vi "Trigger With SubVi.vi"() -> ()   [LabVIEW 2022 SP3]
uses:
  Keithley 24XX Sweep and Acquire Measurements Folder/Keithley 24XX.lvlib
  <instrlib>/Keithley 2182/Keithley 2182.lvlib
panel:
  in  "Enable Current Auto Range (T:Enable)":bool=TRUE
  in  "Current Manual Range (1.0)":dbl=1.0
  out "Measurements":dbl[](array[numeric])
  in  "Integration Rate (5)":dbl=5.0
  in  "Range Value (12)":dbl=12.0
  in  "Voltage Resolution (8)":i32=8
  in  "Measurement (0: Voltage Channel 1) 2":i32(ring) items=["Voltage Channel 1", "Voltage Channel 2", "Temperature Channel 1", "Temperature Channel 2"]
  in  "2182A":T1={"Baud Rate"=9600, "Parity"=0, "Data Bits"=8, "Stop Bits"=10, "Flow Control"=0, "VISA resource name"="SourceMeter2400"} {"Flow Control" items=["None", "XON/XOFF", "RTS/CTS", "XON/XOFF & RTS/CTS", "DTR/DSR", "XON/XOFF & DTR/DSR"]; "Stop Bits" items=["1.0"=10, "1.5"=15, "2.0"=20]; "Data Bits" items=["7"=7, "8"=8]; "Parity" items=["None", "Odd", "Even", "Mark", "Space"]; "Baud Rate" items=["300"=300, "600"=600, "1200"=1200, "2400"=2400, "4800"=4800, "9600"=9600, "19200"=19200]}
  in  "2400":T1={"Baud Rate"=9600, "Parity"=0, "Data Bits"=8, "Stop Bits"=10, "Flow Control"=0, "VISA resource name"="NanoVoltMeter2182"} {"Flow Control" items=["None", "XON/XOFF", "RTS/CTS", "XON/XOFF & RTS/CTS", "DTR/DSR", "XON/XOFF & DTR/DSR"]; "Stop Bits" items=["1.0"=10, "1.5"=15, "2.0"=20]; "Data Bits" items=["7"=7, "8"=8]; "Parity" items=["None", "Odd", "Even", "Mark", "Space"]; "Baud Rate" items=["300"=300, "600"=600, "1200"=1200, "2400"=2400, "4800"=4800, "9600"=9600, "19200"=19200]}
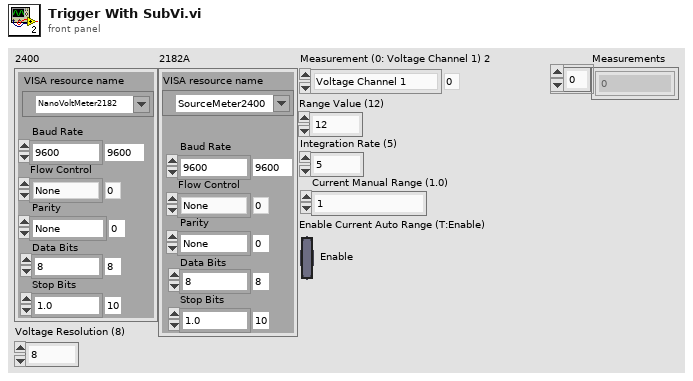
[diagram p1: front panel]
types:
  T1 = cluster{"Baud Rate":u32, "Parity":u16, "Data Bits":u16, "Stop Bits":u16, "Flow Control":u16, "VISA resource name":refnum<visa-resource-name>}
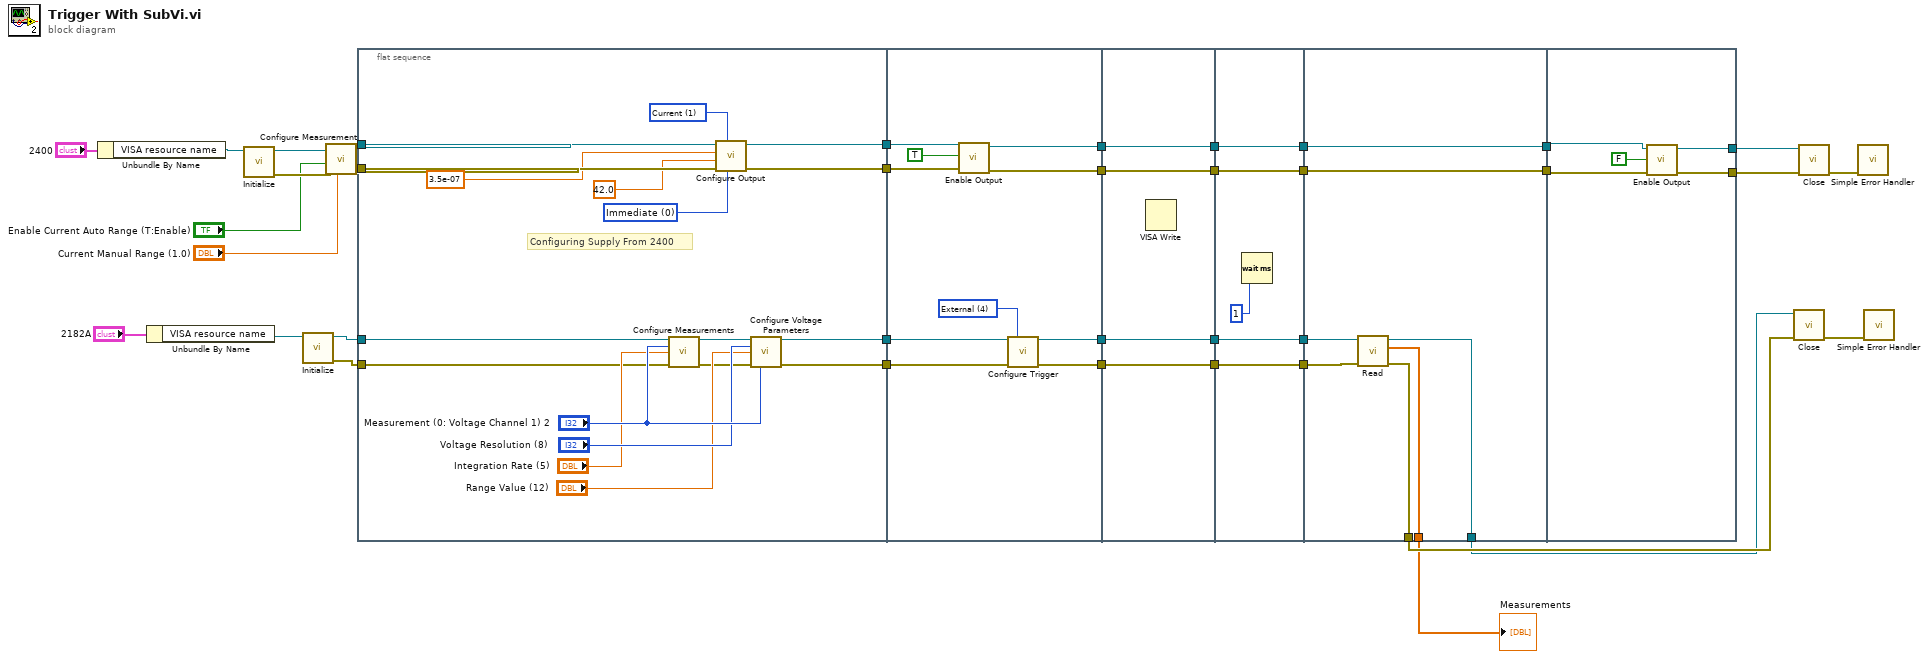
[diagram p0: block diagram]
diagram:
  n1 = Unbundle By Name("2400") -> ("VISA resource name"=w36:refnum<visa-resource-name>)
  n2 = Unbundle By Name("2182A") -> ("VISA resource name"=w32:refnum<visa-resource-name>)
  n3 = call <instrlib>:"Initialize.vi"("VISA resource name"=w36) -> ("error out"=w34:errorcluster, "VISA resource name out"=w35:refnum<visa-resource-name>)  [unwired: 9 in]
  n4 = call <instrlib>:"Initialize.vi"("VISA resource name"=w32) -> ("error out"=w28:errorcluster, "VISA resource name out"=w29:refnum<visa-resource-name>)  [unwired: 9 in]
  n5 = call "Configure Measurement.vi"("Manual Range (1.0)"="Current Manual Range (1.0)", "error in (no error)"=w34, "Enable Auto Range (T:Enable)"="Enable Current Auto Range (T:Enable)", "VISA resource name"=w35) -> ("error out"=w30:errorcluster, "VISA resource name out"=w31:refnum<visa-resource-name>)  [unwired: 6 in]
  n6 = flat-sequence {
    tunnel: w31 -> [w48]
    tunnel: w30 -> [w47]
    tunnel: w29 -> [w46]
    tunnel: w28 -> [w45]
    tunnel: [w44] -> w27
    tunnel: [w43] -> w26
    tunnel: [w42] -> w25
    tunnel: [w41] -> w24
    tunnel: w27 -> [w64]
    tunnel: w26 -> [w63]
    tunnel: w25 -> [w62]
    tunnel: [w61] -> w8
    tunnel: w24 -> [w60]
    tunnel: [w59] -> w6
    tunnel: [w57] -> w4
    tunnel: [w56] -> w2
    tunnel: w8 -> [w69]
    tunnel: [w69] -> w7
    tunnel: w6 -> [w68]
    tunnel: [w68] -> w5
    tunnel: w4 -> [w67]
    tunnel: [w67] -> w3
    tunnel: w2 -> [w66]
    tunnel: [w66] -> w1
    tunnel: w7 -> [w71]
    tunnel: w5 -> [w70]
    tunnel: [w73] -> w23
    tunnel: w3 -> [w73]
    tunnel: [w72] -> w21
    tunnel: w1 -> [w72]
    tunnel: [w71] -> w15
    tunnel: [w70] -> w14
    tunnel: w23 -> [w81]
    tunnel: [w81] -> w22
    tunnel: w21 -> [w80]
    tunnel: [w80] -> w20
    tunnel: w15 -> [w79]
    tunnel: w14 -> [w78]
    tunnel: [w77] -> w13
    tunnel: [w76] -> w12
    tunnel: [w75] -> w11
    tunnel: w22 -> [w83]
    tunnel: w20 -> [w82]
    tunnel: [w85] -> w17
    tunnel: [w84] -> w16
    frame #0 {
      w39 = u16 1 items=["Voltage", "Current"] ("Source Mode  (0: Voltage)")
      w49 = u16 0 items=["Immediate", "Triggered"] ("Output Type  (0: Immediate)")
      # "Configuring Supply From 2400"
      n7 = call <instrlib>:"Configure Measurements.vi"("VISA resource name"=w46, "Measurement (0: Voltage Channel 1)"="Measurement (0: Voltage Channel 1) 2", "Integration Rate (5)"="Integration Rate (5)", "error in (no error)"=w45) -> ("VISA resource name out"=w50:refnum<visa-resource-name>, "error out"=w51:errorcluster)  [unwired: 10 in]
      n8 = call "Configure Output.vi"("Output Type  (0: Immediate)"=w49, "Source Mode  (0: Voltage)"=w39, "error in (no error)"=w47, "Compliance  Level (0.1)"=42.0, "Output Level (0)"=3.5e-07, "VISA resource name"=w48) -> ("error out"=w43:errorcluster, "VISA resource name out"=w44:refnum<visa-resource-name>)  [unwired: 4 in]
      n9 = call <instrlib>:"Configure Voltage Parameters.vi"("VISA resource name"=w50, "Measurement (1: Voltage Channel 1)"="Measurement (0: Voltage Channel 1) 2", "Voltage Resolution (8)"="Voltage Resolution (8)", "Range Value (12)"="Range Value (12)", "error in (no error)"=w51) -> ("VISA resource name out"=w42:refnum<visa-resource-name>, "error out"=w41:errorcluster)  [unwired: 9 in]
    }
    frame #1 {
      w58 = 4 items=["Immediate", "Timer", "Manual", "Bus", "External"] ("Trigger Source (0: Immediate)")
      n10 = call "Enable Output.vi"("error in (no error)"=w63, "Enable Output (T: Enable)"=TRUE, "VISA resource name"=w64) -> ("error out"=w56:errorcluster, "VISA resource name out"=w57:refnum<visa-resource-name>)  [unwired: 7 in]
      n11 = call <instrlib>:"Configure Trigger.vi"("VISA resource name"=w62, "Trigger Source (0: Immediate)"=w58, "error in (no error)"=w60) -> ("VISA resource name out"=w61:refnum<visa-resource-name>, "error out"=w59:errorcluster)  [unwired: 11 in]
    }
    frame #2 {
      n12 = VISA Write() -> ()  [unwired: 3 in, 3 out]
    }
    frame #3 {
      n13 = Wait (ms)(milliseconds to wait=u32 1 ("millisecond timer value")) -> ()  [unwired: 1 out]
    }
    frame #4 {
      n14 = call <instrlib>:"Read.vi"("error in (no error)"=w78, "VISA resource name"=w79) -> ("error out"=w77:errorcluster, "Measurements"=w75:dbl[], "VISA resource name out"=w76:refnum<visa-resource-name>)  [unwired: 6 in, 1 out]
    }
    frame #5 {
      n15 = call "Enable Output.vi"("error in (no error)"=w82, "Enable Output (T: Enable)"=FALSE, "VISA resource name"=w83) -> ("error out"=w85:errorcluster, "VISA resource name out"=w84:refnum<visa-resource-name>)  [unwired: 7 in]
    }
  }
  n16 = call <instrlib>:"Close.vi"("error in (no error)"=w13, "VISA resource name"=w12) -> ("error out"=w18:errorcluster)  [unwired: 9 in]
  n17 = call <instrlib>:"Close.vi"("error in (no error)"=w17, "VISA resource name"=w16) -> ("error out"=w19:errorcluster)  [unwired: 9 in]
  n18 = call <vilib>:"Simple Error Handler.vi"("error in (no error)"=w19) -> ()  [unwired: 4 in, 5 out]
  n19 = call <vilib>:"Simple Error Handler.vi"("error in (no error)"=w18) -> ()  [unwired: 4 in, 5 out]
  "Measurements" <- w11
